vi "Write New Data Msg.vi"(10 "Calling Actor.lvlib:New Data Msg.lvclass":refnum<class "New Data Msg.lvclass">, 11 "Calling Actor in":refnum<class "Calling Actor.lvclass">) -> (3 "Calling Actor out":refnum<class "Calling Actor.lvclass">)   [LabVIEW 2018, in "Calling Actor.lvlib" / "Calling Actor.lvclass"]
uses:
  Calling Actor.lvclass
  Calling Actor Messages/New Data Msg/New Data Msg.lvclass
  Calling Actor.lvclass/Calling Actor.ctl
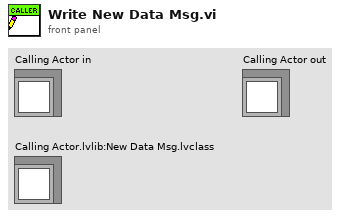
[diagram p1: front panel]
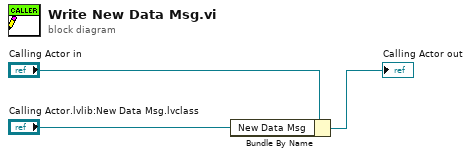
[diagram p0: block diagram]
diagram:
  n1 = Bundle By Name(cluster="Calling Actor in", "New Data Msg"="Calling Actor.lvlib:New Data Msg.lvclass") -> (→"Calling Actor out":refnum<class "Calling Actor.lvclass">)
